vi "2P結束.vi"(1 "Array":dbl[][](array[numeric]), 2 "String 2":string, 3 "String":string) -> (4 "onemore 2":bool, 5 "final 2":bool)   [LabVIEW 2014]
panel:
  in  "final":bool
  out "Array 2":dbl[][](array[numeric])
  out "String 4":string
  out "String 3":string
  in  "onemore":bool
  # "分數:"
  # "害死青蛙數:"
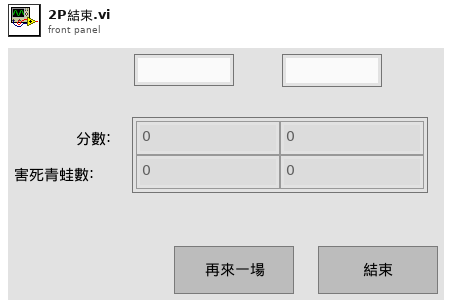
[diagram p1: front panel]
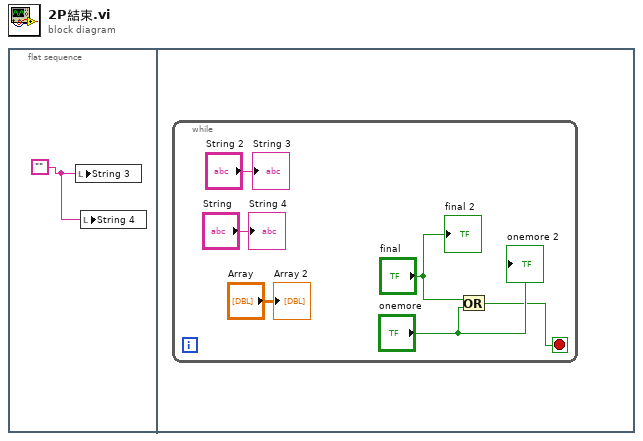
[diagram p0: block diagram]
diagram:
  n1 = flat-sequence {
    frame #0 {
      w1 = ""
      n2 = local write "String 3"(w1) -> ()
      n3 = local write "String 4"(w1) -> ()
    }
    frame #1 {
      n4 = while {
        stop <- w2 stop-if-true
        n5 = Or(x="final", y="onemore") -> (x .or. y?=w2:bool)
        "String 3" <- "String 2"
        "String 4" <- "String"
        "Array 2" <- "Array"
        "final 2" <- "final"
        "onemore 2" <- "onemore"
      }
    }
  }
